vi "power2deg_steps2.vi"(8 "Max_power":dbl, 9 "Min_power":dbl, 10 "Min_angle":dbl, 11 "Power":dbl) -> (2 "Steps":i32, 3 "Deg":dbl)   [LabVIEW 2015]
panel:
  in  "Offset":i32
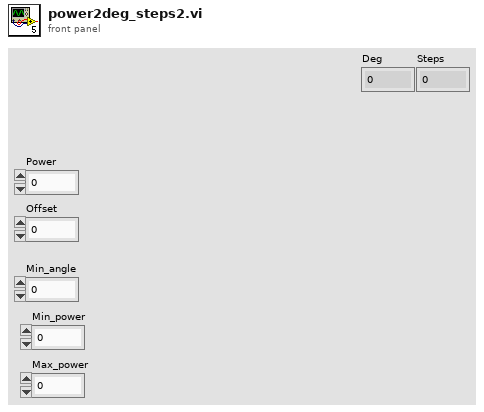
[diagram p1: front panel]
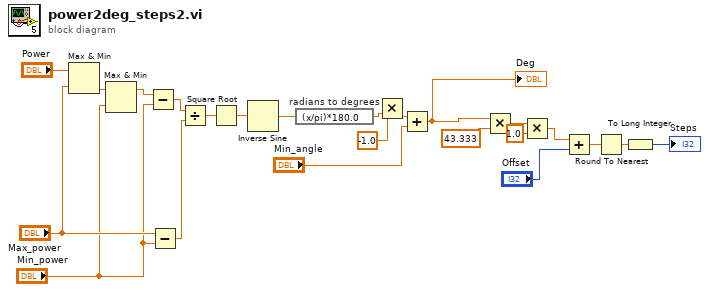
[diagram p0: block diagram]
diagram:
  n1 = Max & Min(x="Power", y="Max_power") -> (min(x,y)=w3:dbl)  [unwired: 1 out]
  n2 = Max & Min(x=w3, y="Min_power") -> (max(x,y)=w1:dbl)  [unwired: 1 out]
  n3 = Subtract(x=w1, y="Min_power") -> (x-y=w23:dbl)
  n4 = Subtract(x="Max_power", y="Min_power") -> (x-y=w22:dbl)
  n5 = Divide(x=w23, y=w22) -> (x/y=w21:dbl)
  n6 = Square Root(x=w21) -> (sqrt(x)=w20:dbl)
  n7 = Inverse Sine(1:w20) -> (0:w19:dbl)
  n8 = expression code="(x/pi)*180.0" "radians to degrees"(w19) -> (w10:dbl)
  n9 = Multiply(x=-1.0, y=w10) -> (x*y=w7:dbl)
  n10 = Add(x=w7, y="Min_angle") -> (x+y=w8:dbl)
  "Deg" <- w8
  n11 = Multiply(x=w8, y=43.333) -> (x*y=w17:dbl)
  n12 = Multiply(x=w17, y=1.0) -> (x*y=w15:dbl)
  n13 = Add(x=w15, y="Offset") -> (x+y=w13:dbl)
  n14 = Round To Nearest(number=w13) -> (nearest integer value=w12:dbl)
  n15 = To Long Integer(number=w12) -> (32bit integer=→"Steps":i32)
